vi "Get Data.vi"(7 "timeout ms (25000)":i32, 8 "Error In":errorcluster, 11 "connection ID":refnum<k16>) -> (0 "Error Out":errorcluster, 2 "Data output":T1, 3 "connection ID out":refnum<k16>)   [LabVIEW 2016, in "MKR1000.lvlib"]
doc: "Manage the string received by MKR1000 to be plotted properly.\n\nNOTE:\nThe MKR1000 VI Library uses UDP. UDP is a connectionless protocol. With the term \"connection\" is intended that MKR1000 gives back an ACKnoledgment packet for each command sent. If no packet is returned (MKR1000 not connected to the net, out of range, etc.), the command is intended LOST and the VIs attempts to send the command again few times before returning Error 5000"
uses:
  MKR1000.lvlib
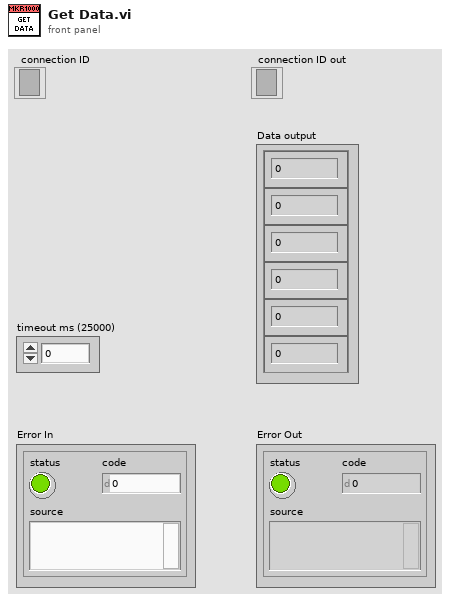
[diagram p1: front panel]
types:
  T1 = cluster{"Numeric Control":sgl, "Numeric Control":sgl, "Numeric Control":sgl, "Numeric Control":sgl, "Numeric Control":sgl, "Numeric Control":sgl}
  T2 = cluster{"[0]":sgl, "[1]":sgl, "[2]":sgl, "[3]":sgl, "[4]":sgl, "[5]":sgl}
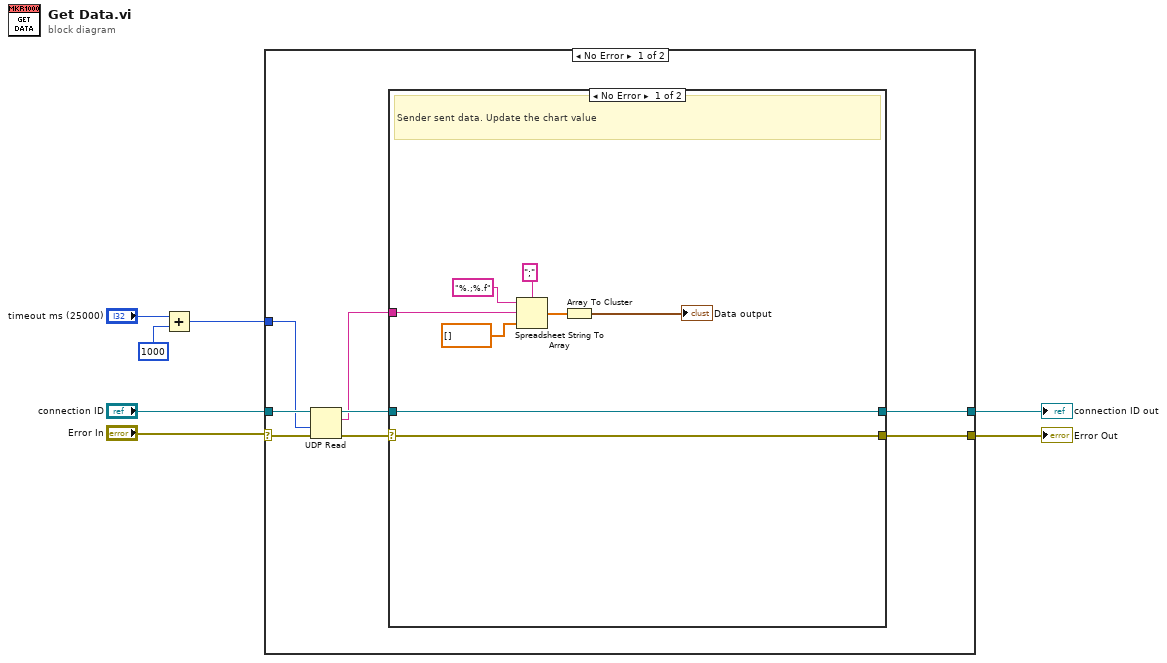
[diagram p0: block diagram]
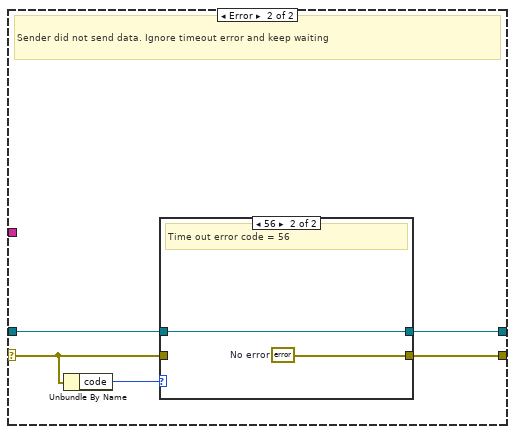
[diagram p2: hidden frame]
diagram:
  n1 = Add(x="timeout ms (25000)", y=1000) -> (x+y=w1:i32)
  n2 = case shown="No Error" "Error In" {
    selector: "Error In" -> [w15 w34]
    tunnel: [w13 w34] -> w6
    tunnel: "connection ID" -> [w12 w33]
    tunnel: w1 -> [w8 _]
    tunnel: [w9 w33] -> w4
    frame No Error {
      n3 = UDP Read(connection ID=w12, timeout ms (25000)=w8, 8:w15) -> (data out=w10:string, error out=w14:errorcluster, 3:w11:refnum<k16>)  [unwired: 3 out]
      n4 = case shown="No Error" w14 {
        selector: w14 -> [w22 w26]
        tunnel: [w22 w27] -> w13
        tunnel: w11 -> [w23 w25]
        tunnel: [w23 w24] -> w9
        tunnel: w10 -> [w19 _]
        frame No Error {
          # "Sender sent data. Update the chart value"
          n5 = Spreadsheet String To Array(delimiter (Tab)=";", format string="%.;%.f", spreadsheet string=w19, array type (2D Dbl)=sgl[] []) -> (array=w18:sgl[])
          n6 = Array To Cluster(array=w18) -> (cluster=→"Data output":T2)
        }
        frame Error {
          # "Sender did not send data. Ignore timeout error and keep waiting"
          n7 = Unbundle By Name(w26) -> ("code"=w28:i32)
          n8 = case shown="56" w28 {
            tunnel: w26 -> [w30 _]
            tunnel: [w30 w32] -> w27
            tunnel: w25 -> [w29 w31]
            tunnel: [w29 w31] -> w24
            frame Default {
            }
            frame 56 {
              w32 = errorcluster {"status"=FALSE, "code"=0, "source"=""}  # No error
              # "Time out error code = 56"
            }
          }
        }
      }
    }
    frame Error {
    }
  }
  "Error Out" <- w6
  "connection ID out" <- w4
